vi "PH_Timing.set GD Stati to GUI.vi"(0 "VI in":refnum<vi>, 5 "error in (no error)":errorcluster) -> (14 "VI out":refnum<vi>, 19 "error out":errorcluster)   [LabVIEW 2014, in "PH_Timing.lvlib"]
uses:
  PH_Timing.lvlib
  PH_Common/PH_Common.lvlib
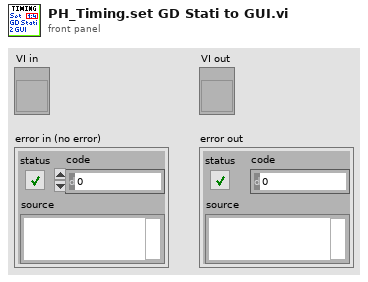
[diagram p1: front panel]
types:
  T1 = typedef "PH_Timing.lvlib/PH_Timing.i attribute.ctl" = cluster{"Sequencer":cluster{"linked?":bool, "Proc State":string, "Ref State":refnum<vi>}, "Gate Generator":cluster{"GD":cluster{"Device Status":T2, "linked?":bool}, "Settings":T3, "GUI Ref":refnum<vi>}, "Interlock Bypass":cluster{"Instancename":string, "Switch linked?":bool, "Device Status":T2, "Ref Status":refnum<vi>}, "Roughtuner":cluster{"Settings":T4, "GUI Ref":refnum<vi>, "GD":cluster{"Device Status":T2, "linked?":bool}}, "0,5Hz Gater":cluster{"Settings":T5, "GUI Ref":refnum<vi>, "GD":cluster{"Device Status":T2, "linked?":bool}}, "Slow Trigger":cluster{"Settings":T6, "GUI Ref":refnum<vi>, "Service ID Delay":i32, "Service ID Ext Trig":i32, "Wanted Settings":T6}, "Timing Mode":cluster{"Mode":T7, "GUI Ref":refnum<vi>, "Service ID T2":i32, "Service ID Mode":i32, "Wanted Mode":T7}, "ns Generator":cluster{"Settings":T8, "ns Generator Settings":refnum<vi>, "GD":cluster{"Device Status":T2, "linked?":bool}}, "Phase FEs":cluster{"Settings":T11, "GUI Ref":refnum<vi>, "Service ID Phase":i32, "Wanted Settings":T11}, "GD GUI Refs":refnum<vi>[], "Heads":T12[], "GUI Ref Delete":refnum<vi>}
  T2 = typedef "PH_StatusHandler.lvlib/PH_StatusHandler.Status.ctl" = i16
  T3 = typedef "PH_Timing.lvlib/PH_Timing.GateGen.ctl" = cluster{"Instance":string, "Channel Gate":i32, "Channel T2":i32, "Width Gate":dbl, "Width T2":dbl, "Delay Gate":dbl, "Delay T2":dbl, "Gate activ":bool, "T2 activ":bool, "System Mode":enum16{"Normal", "Single", "Burst", "Duty Cycle"}}
  T4 = typedef "PH_Timing.lvlib/PH_Timing.Roughtuner.ctl" = cluster{"Instance":string, "Phase PHELIX / UNILAC":cluster{"Channel":u16, "relative to":u16, "Delay [ms]":dbl}, "Pulse Length":cluster{"Channel":u16, "relative to":u16, "Delay [ms]":dbl}, "Trigger":cluster{"externally?":bool, "Rate [Hz]":dbl}}
  T5 = typedef "PH_Timing.lvlib/PH_Timing.0.5HzGater.ctl" = cluster{"Instance":string, "Channel ns FE Delay":i32, "Channel 0.5Hz":i32, "Width ns FE Delay":dbl, "Width 0.5Hz":dbl, "Delay ns FE Delay":dbl, "Delay 0.5Hz":dbl, "ns FE Delay active":bool, "0.5Hz activ":bool, "ns FE Delay inverted":bool, "0.5Hz inverted":bool}
  T6 = typedef "PH_Timing.lvlib/PH_Timing.Slow Trigger Settings.ctl" = cluster{"Delay":dbl, "externally triggered?":bool}
  T7 = typedef "PH_Timing.lvlib/PH_Timing.Timing Mode.ctl" = cluster{"T2":i16, "Modeselector":enum32{"10 Hz", "0.5 Hz", "Shot"}}
  T8 = typedef "PH_Timing.lvlib/PH_Timing.ns Generator.ctl" = cluster{"Instance":string, "Phase fs / ns FE":cluster{"Channel":T9, "Settings":T10}}
  T9 = typedef "Stanford Research DG645 - Driver.lvlib/Channel.ctl" = i32
  T10 = typedef "PH_SRDG645.lvlib/PH_SRDG645.Channel Settings.ctl" = cluster{"Delay [s]":dbl, "relative to":i32}
  T11 = typedef "PH_Timing.lvlib/PH_Timing.Phase FEs.ctl" = cluster{"Phase":dbl}
  T12 = typedef "PH_Timing.lvlib/PH_Timing.PU Data.ctl" = cluster{"linked?":bool, "Data":T13, "GD":cluster{"Device Status":T2, "linked?":bool}, "GUI Ref":refnum<vi>, "PU":T14}
  T13 = typedef "PH_Timing.lvlib/PH_Timing.PU Info.ctl" = cluster{"Act CH?":bool, "GD":string, "CH":i32, "Delay":dbl, "active":bool, "in Use?":bool}
  T14 = typedef "PH_PP_Common.lvlib/PH_PP_Common.PUs.ctl" = enum16{"no Info", "PA-19mm-1", "PA-19mm-2", "PA-45mm-PILC", "PA-45mm-MAIN", "MA-PU-1", "MA-PU-2", "MA-PU-3", "MA-PU-4", "MA-PU-5", "MA-PU-6", "MA-FR", "MA-PILC", "PA-45mm-DP"}
  T15 = cluster{"GD":cluster{"Device Status":T2, "linked?":bool}, "Settings":T3, "GUI Ref":refnum<vi>}
  T16 = cluster{"Settings":T4, "GUI Ref":refnum<vi>, "GD":cluster{"Device Status":T2, "linked?":bool}}
  T17 = cluster{"Settings":T5, "GUI Ref":refnum<vi>, "GD":cluster{"Device Status":T2, "linked?":bool}}
  T18 = cluster{"Settings":T8, "ns Generator Settings":refnum<vi>, "GD":cluster{"Device Status":T2, "linked?":bool}}
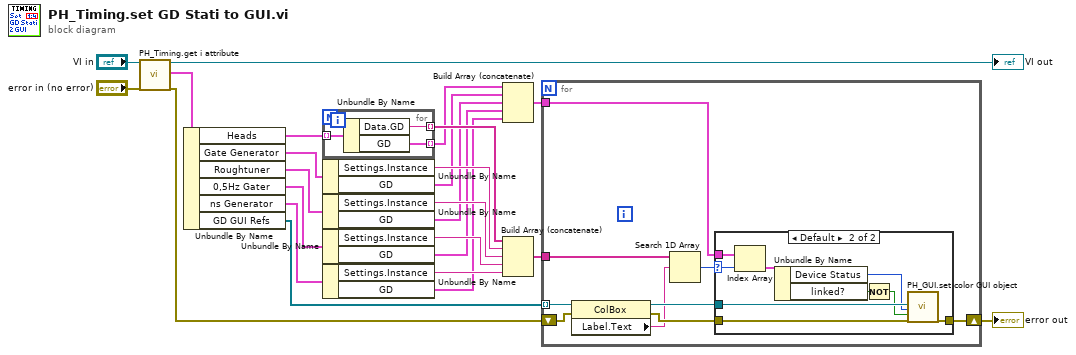
[diagram p0: block diagram]
diagram:
  n1 = call "PH_Timing.get i attribute.vi"("i ref in"="VI in", "error in (no error)"="error in (no error)") -> ("i ref out"=→"VI out":refnum<vi>, "i attribute"=w20:T1, "error out"=w22:errorcluster)  [unwired: 15 in]
  n2 = Unbundle By Name(w20) -> ("Heads"=w1:T12[], "Gate Generator"=w17:T15, "Roughtuner"=w16:T16, "0,5Hz Gater"=w15:T17, "ns Generator"=w14:T18, "GD GUI Refs"=w18:refnum<vi>[])
  n3 = for {
    tunnel: w1 -> [w27] mode=indexing
    tunnel: [w26] -> w3 mode=indexing
    tunnel: [w25] -> w8 mode=indexing
    n4 = Unbundle By Name(w27) -> ("Data.GD"=w25:string, "GD"=w26:cluster{"Device Status":T2, "linked?":bool})
  }
  n5 = Unbundle By Name(w17) -> ("Settings.Instance"=w12:string, "GD"=w4:cluster{"Device Status":T2, "linked?":bool})
  n6 = Unbundle By Name(w16) -> ("Settings.Instance"=w11:string, "GD"=w5:cluster{"Device Status":T2, "linked?":bool})
  n7 = Unbundle By Name(w15) -> ("Settings.Instance"=w10:string, "GD"=w6:cluster{"Device Status":T2, "linked?":bool})
  n8 = Unbundle By Name(w14) -> ("Settings.Instance"=w9:string, "GD"=w7:cluster{"Device Status":T2, "linked?":bool})
  n9 = Build Array (concatenate)(w3, w4, w5, w6, w7) -> (w2:cluster{"Device Status":T2, "linked?":bool}[])
  n10 = Build Array (concatenate)(w8, w12, w11, w10, w9) -> (w13:string[])
  n11 = for {
    tunnel: w18 -> [w35] mode=indexing
    shift-right: [w36] -> w19
    shift-left: w22 -> [w33]
    tunnel: w13 -> [w31]
    tunnel: w2 -> [w29]
    n12 = property class="ColBox"(reference=w35, error in=w33) -> (reference out=w34:refnum<vi>, error out=w32:errorcluster, "Label.Text"=w30:string)
    n13 = Search 1D Array(1D array=w31, element=w30) -> (index of element=w28:i32)  [unwired: 1 in]
    n14 = case shown="Default" w28 {
      selector: w28 -> [_ w42]
      tunnel: [w37 w46] -> w36
      tunnel: w34 -> [_ w45]
      tunnel: w32 -> [w37 w44]
      tunnel: w29 -> [_ w43]
      frame -1 {
      }
      frame Default {
        n15 = Index Array(array=w43, index=w42) -> (element=w41:cluster{"Device Status":T2, "linked?":bool})
        n16 = Unbundle By Name(w41) -> ("Device Status"=w40:T2, "linked?"=w39:bool)
        n17 = Not(x=w39) -> (.not. x?=w38:bool)
        n18 = call "PH_GUI.set color GUI object.vi"("GUI object Ref"=w45, "State"=w40, "Blinking? (false)"=w38, "error in (no error)"=w44) -> ("error out"=w46:errorcluster)  [unwired: 15 in]
      }
    }
  }
  "error out" <- w19
